vi "OnOffGenParametrFromSTAR (SubVI).vi"(4 "VChGen":refnum<vi>, 6 "fGEN1":refnum<vi>, 7 "Fa":refnum<vi>, 8 "FGen":refnum<vi>, 9 "AutoA":refnum<vi>, 10 "AutoB":refnum<vi>, 11 "Fb":refnum<vi>) -> ()   [LabVIEW 2017]
uses:
  st_str Global.vi
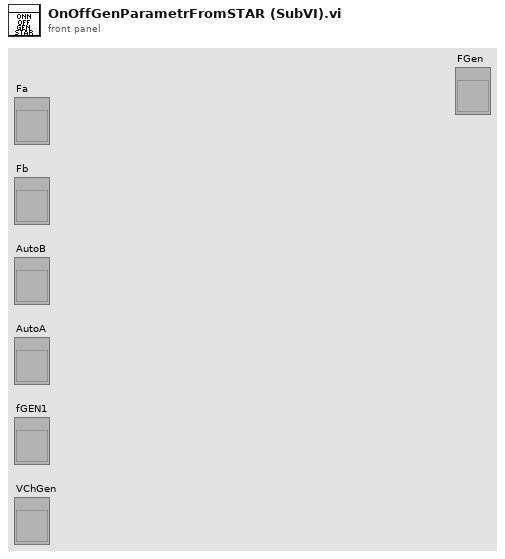
[diagram p1: front panel]
types:
  T1 = enum8{"Enabled", "Disabled", "Disabled and Grayed Out"}
  T2 = typedef "A5000_param.ctl" = cluster{"ChannelA":cluster{"Enabled":bool, "Coupling":i16, "Range":u16, "Analogue Offset":sgl}, "ChannelB":cluster{"Enabled":bool, "Coupling":i16, "Range":u16, "Analogue Offset":sgl}, "Trigger":cluster{"Trigger Enabled":bool, "Trigger Source":enum16{"Channel A", "Channel B", "Channel C", "Channel D", "Ext."}, "Trigger Threshold (volts)":dbl, "Trigger Direction":u16, "Trigger Delay (samples)":u32, "Auto Trigger Time (ms)":i16}, "MaxADCvalue":i16, "handle":i16, "Acquisition":cluster{"preTriggerSamples":i32, "postTriggerSamples":i32, "timebase":u32, "Down-Sample Mode":u32, "Down Sample Ratio":u32}, "Device Info":cluster{"Driver Version":string, "USB Version":string, "Hardware":string, "Variant":string, "Batch and Serial":string, "Cal Date":string, "Kernel Version":string, "Digital HW Version":string, "Analogue HW Version":string, "MSO":bool, "Number of channels":i16}, "Properties":cluster{"Sample Frequency":sgl, "Sample Rate":sgl, "Max Samples Available":i32, "Number of Samples":u32, "Total Capture Time (sec) ":sgl, "Max Total Capture Time Available (sec)":sgl}, "Resolution":i32, "EmulateV":bool, "General AWG Settings":cluster{"Peak-to-Peak Voltage (microvolts)":u32, "Offset Voltage (microvolts)":i32, "Wave Type":u32, "Sweep Type":u32, "Shots":u32, "Sweeps":u32, "Trigger Type":u32, "Trigger Source":u32, "Ext. Threshold (ADC count)":i16, "White Noise/PRBS":u32}, "Standard Waveform Settings":cluster{"Start Frequency":dbl, "Stop Frequency":dbl, "Increment":dbl, "Dwell Time (seconds)":dbl}, "Arbitrary Waveform Settings":cluster{"Arbirary waveform file path":path, "Index Mode":u32}, "AutoDiapChA":bool, "AutoDiapChB":bool}
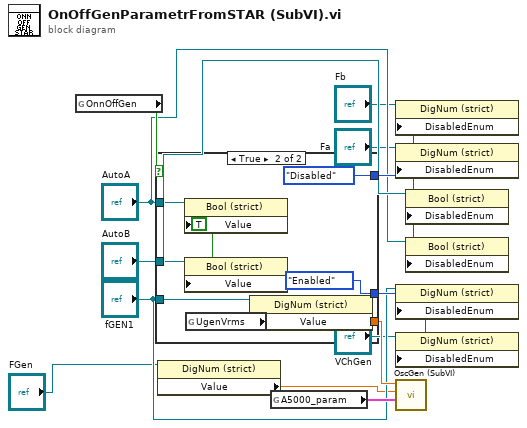
[diagram p0: block diagram]
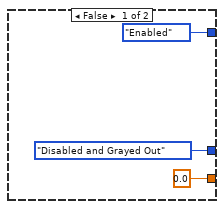
[diagram p2: hidden frame]
diagram:
  n1 = global read "st_str Global.vi" "OnnOffGen"() -> (w9:bool)
  n2 = case shown="True" w9 {
    tunnel: [T1."Disabled and Grayed Out" ("Disabled") T1."Enabled" ("Disabled")] -> w10
    tunnel: [T1."Enabled" ("Disabled") T1."Disabled" ("Disabled")] -> w11
    tunnel: [0.0 ("UgenVrms") w20] -> w13
    tunnel: "AutoB" -> [_ w19]
    tunnel: "AutoA" -> [_ w18]
    tunnel: "fGEN1" -> [_ w17]
    frame False {
    }
    frame True {
      w23 = TRUE ("AutoFindFreqChB")
      n3 = property on="Property Node" class="Bool (strict)"(reference=w18, "Value"=w23) -> ()  [unwired: 1 in, 2 out]
      n4 = property on="Property Node" class="Bool (strict)"(reference=w19, "Value"=w23) -> ()  [unwired: 1 in, 2 out]
      n5 = global read "st_str Global.vi" "UgenVrms"() -> (w20:dbl)
      n6 = property class="DigNum (strict)"(reference=w17, "Value"=w20) -> ()  [unwired: 1 in, 2 out]
    }
  }
  n7 = property class="DigNum (strict)"(reference="FGen") -> ("Value"=w1:dbl)  [unwired: 1 in, 2 out]
  n8 = global read "st_str Global.vi" "A5000_param"() -> (w12:T2)
  n9 = property on="Property Node" class="DigNum (strict)"(reference="Fb", "DisabledEnum"=w11) -> ()  [unwired: 1 in, 2 out]
  n10 = property on="Property Node" class="DigNum (strict)"(reference="Fa", "DisabledEnum"=w11) -> ()  [unwired: 1 in, 2 out]
  n11 = property on="Property Node" class="DigNum (strict)"(reference="fGEN1", "DisabledEnum"=w10) -> ()  [unwired: 1 in, 2 out]
  n12 = property on="Property Node" class="DigNum (strict)"(reference="VChGen", "DisabledEnum"=w10) -> ()  [unwired: 1 in, 2 out]
  n13 = call "OscGen (SubVI).vi"("A5000_param_out"=w12, "Frequency,kHz"=w1, "UgenVrms"=w13) -> ()  [unwired: 8 in, 1 out]
  n14 = property on="Property Node" class="Bool (strict)"(reference="AutoB", "DisabledEnum"=w11) -> ()  [unwired: 1 in, 2 out]
  n15 = property on="Property Node" class="Bool (strict)"(reference="AutoA", "DisabledEnum"=w11) -> ()  [unwired: 1 in, 2 out]
